vi "savedata.vi"() -> ()   [LabVIEW 2011]
uses:
  <vilib>/Utility/file.llb/Write To Spreadsheet File (I64).vi
panel:
  in  "Record button":bool
  out "Waveform Chart":T1(graph)
  in  "Log file":path
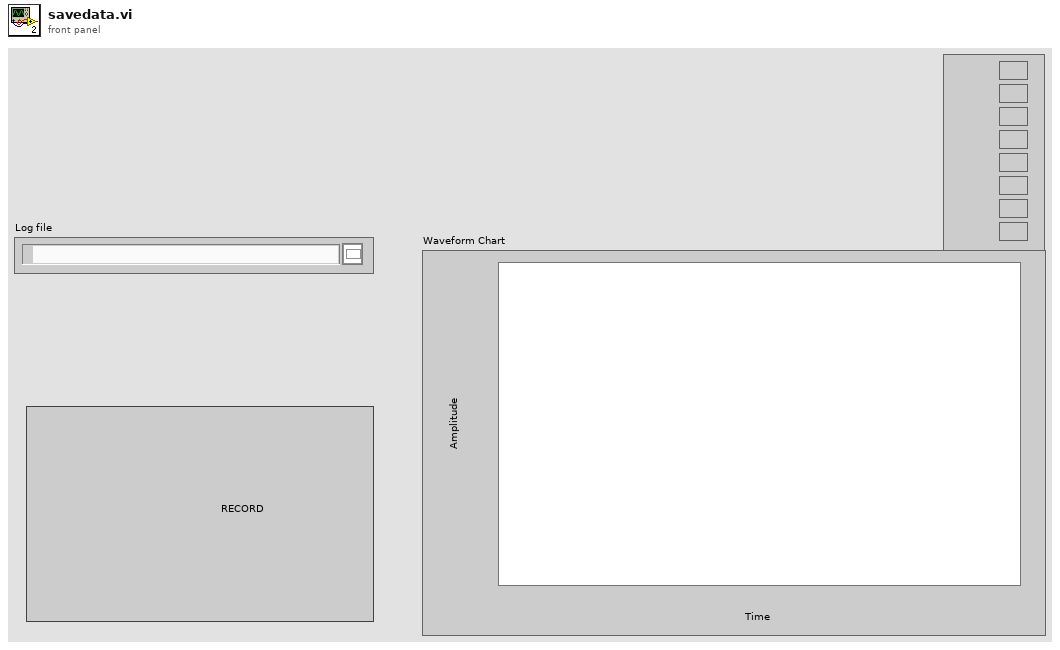
[diagram p1: front panel]
types:
  T1 = cluster{"[0]":u16, "[1]":u16, "[2]":u16, "[3]":u16, "[4]":u16, "[5]":u16, "[6]":u16, "[7]":u16, "[8]":u16}
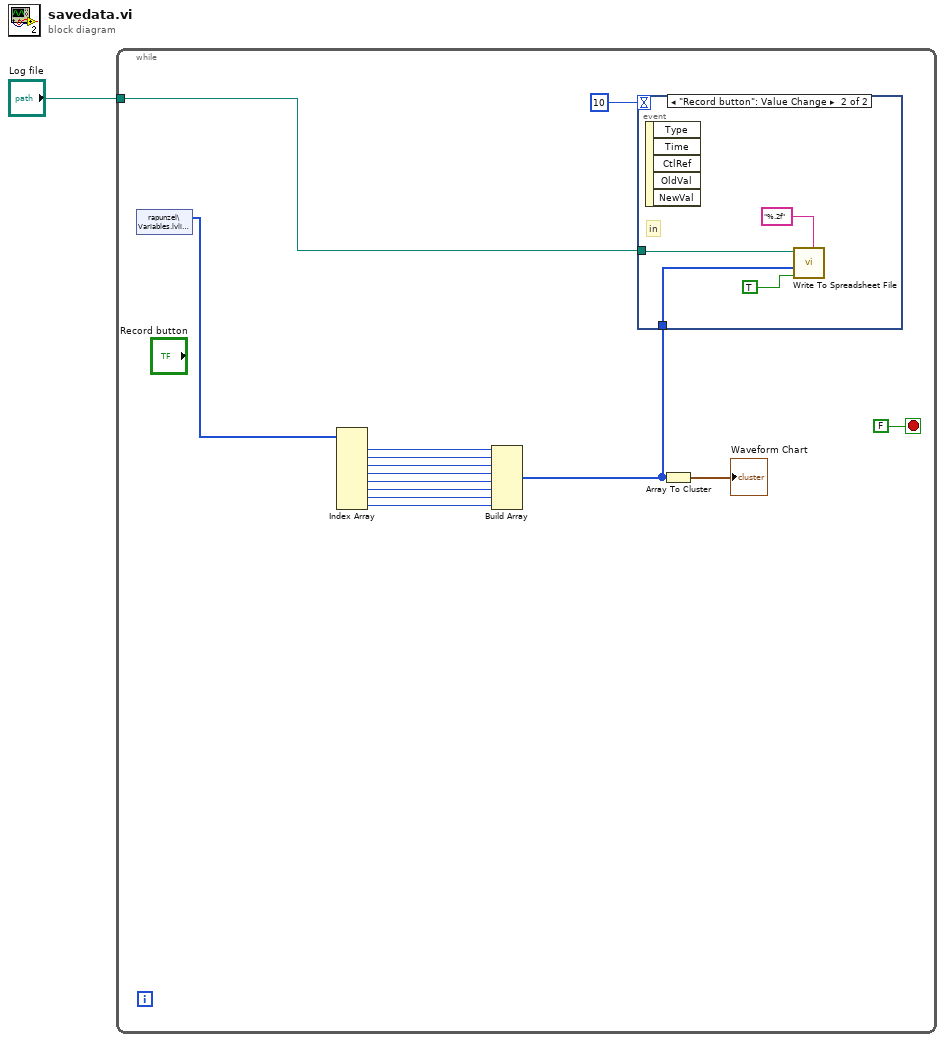
[diagram p0: block diagram]
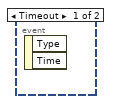
[diagram p2: hidden frame]
diagram:
  n1 = while {
    tunnel: "Log file" -> [w14]
    stop <- FALSE stop-if-true
    n2 = shared-variable "rapunzel\\Variables.lvlib\\AI"() -> (w12:u16[])  [unwired: 1 in, 1 out]
    n3 = Index Array(array=w12) -> (element #1=w5:u16, element #2=w6:u16, element #3=w7:u16, element #4=w8:u16, element #5=w9:u16, element #6=w10:u16, element #7=w11:u16, element #8=w3:u16)  [unwired: 8 in]
    n4 = Build Array(w5, w6, w7, w8, w9, w10, w11, w3) -> (w2:u16[])
    n5 = event shown="[1] \"Record button\": Value Change" {
      selector: _ -> [_ _]
      dyn-events: _ -> [_ _]
      timeout: 10 -> [_ _]
      tunnel: w14 -> [_ w17]
      tunnel: w2 -> [_ w16]
      event Timeout {
        n6 = event-data() -> ()  [unwired: 1 in, 2 out]
      }
      event "Record button": Value Change {
        # "in"
        n7 = event-data() -> ()  [unwired: 1 in, 5 out]
        n8 = call-poly <vilib>:"Write To Spreadsheet File.vi"("format (%d)"="%.2f" ("format (%.3f)"), "append to file? (new file:F)"=TRUE, "1D data"=w16, "file path (dialog if empty)"=w17) -> ()  [unwired: 4 in, 1 out]
      }
    }
    n9 = Array To Cluster(array=w2) -> (cluster=→"Waveform Chart":T1)
  }
